vi "MGCC_StaEst_opal_RT_convertPnode.vi"(10 "cluster":T1) -> (2 "P_node":T1)   [LabVIEW 2016]
doc: "-----------------------------------------------------------------------------------------------------------------------\nCopyright <2019> <The University of Tennessee at Knoxville and the University of Tennessee Research Foundation>\nThis software is released under BSD-3 \nhttps://opensource.org/licenses/BSD-3-Clause \nAdditional license options available at https://utrf.tennessee.edu/industry/sample-agreements/\n-----------------------------------------------------------------------------------------------------------------------"
uses:
  Model Management/Global_MdlMgmt.vi
  <vilib>/imath/engines/lvmath2/RunTimeEngine/IndexRead/NIMS M($,S).vi
  <instcachedir>/0/NIMS M($,S)_3E5749BBB62E49528D4765A77F1F6D98.lvgen/NIMS M($,S)_3E5749BBB62E49528D4765A77F1F6D98_001.vi
  <vilib>/imath/engines/lvmath2/RunTimeEngine/BuiltInFunctions/length/NIMS_length(GV).vi
  <instcachedir>/0/NIMS_length(GV)_08A3D13377FD4E4B96F5795FBF3698FA.lvgen/NIMS_length(GV)_08A3D13377FD4E4B96F5795FBF3698FA_001.vi
  <vilib>/imathl/engines/lvmath/Functions/Error Handling/Create Error.vi
  <vilib>/imath/engines/lvmath2/RunTimeEngine/RangeToken/NIMS_Range_R3 - Integer.vi
  <instcachedir>/0/NIMS_Range_R3 - Integer_A435E2FF893B4C718FD5055FE39FE2F6.lvgen/NIMS_Range_R3 - Integer_A435E2FF893B4C718FD5055FE39FE2F6_000.vi
  <vilib>/imath/engines/lvmath2/RunTimeEngine/CommandStatement/MC_CommandStatement_break.vi
  <vilib>/imath/engines/lvmath2/RunTimeEngine/IndexRead/NIMS V(S).vi
  <instcachedir>/0/NIMS V(S)_0488751826AF41519A22953C041130DC.lvgen/NIMS V(S)_0488751826AF41519A22953C041130DC_000.vi
  <vilib>/imath/engines/lvmath2/RunTimeEngine/IndexReplace/NIMS M(S,$)=V.vi
  <instcachedir>/0/NIMS M(S,$)=V_BCCFA522A894489B8FA760383D74A164.lvgen/NIMS M(S,$)=V_BCCFA522A894489B8FA760383D74A164_001.vi
  <instcachedir>/0/NIMS M($,S)_3E5749BBB62E49528D4765A77F1F6D98.lvgen/NIMS M($,S)_3E5749BBB62E49528D4765A77F1F6D98_000.vi
  <instcachedir>/0/NIMS_length(GV)_08A3D13377FD4E4B96F5795FBF3698FA.lvgen/NIMS_length(GV)_08A3D13377FD4E4B96F5795FBF3698FA_000.vi
  <vilib>/imath/engines/lvmath2/RunTimeEngine/IndexRead/NIMS M(S,S).vi
  <instcachedir>/0/NIMS M(S,S)_AC51E74150A542F7991B9634C66F3096.lvgen/NIMS M(S,S)_AC51E74150A542F7991B9634C66F3096_000.vi
  <vilib>/imath/engines/lvmath2/RunTimeSupport/NIMS_Error if Not Equal.vi
  <instcachedir>/0/NIMS_Error if Not Equal_43252A79AD05436189442EC0C5E5AB8A.lvgen/NIMS_Error if Not Equal_43252A79AD05436189442EC0C5E5AB8A_000.vi
  <vilib>/imath/engines/lvmath2/RunTimeEngine/ErrorHandling/NIMS_Create Error From Enums.vi
  <vilib>/imath/engines/lvmath2/RunTimeEngine/IndexRead/NIMS M(S,$).vi
  <instcachedir>/0/NIMS M(S,$)_F24F360562DE41D8BE234322A2E15C65.lvgen/NIMS M(S,$)_F24F360562DE41D8BE234322A2E15C65_001.vi
  <vilib>/imath/engines/lvmath2/RunTimeEngine/NodeEndStatement/NIMS_NodeEndStatement_Output.vi
  <instcachedir>/0/NIMS_NodeEndStatement_Output_53EC0D466D134D7ABD903AC30B43404B.lvgen/NIMS_NodeEndStatement_Output_53EC0D466D134D7ABD903AC30B43404B_003.vi
  <vilib>/imath/engines/lvmath2/RunTimeEngine/ErrorHandling/NIMS_Finalize Error.vi
panel:
  out "Slack_bus":dbl[](array[numeric])
  out "element":dbl
  out "f_MGCC_OnliTopoIden_EnergizedMatrix":dbl[](array[numeric])
  out "error out":errorcluster
  out "p_node 2":cdb[][](array[numeric])
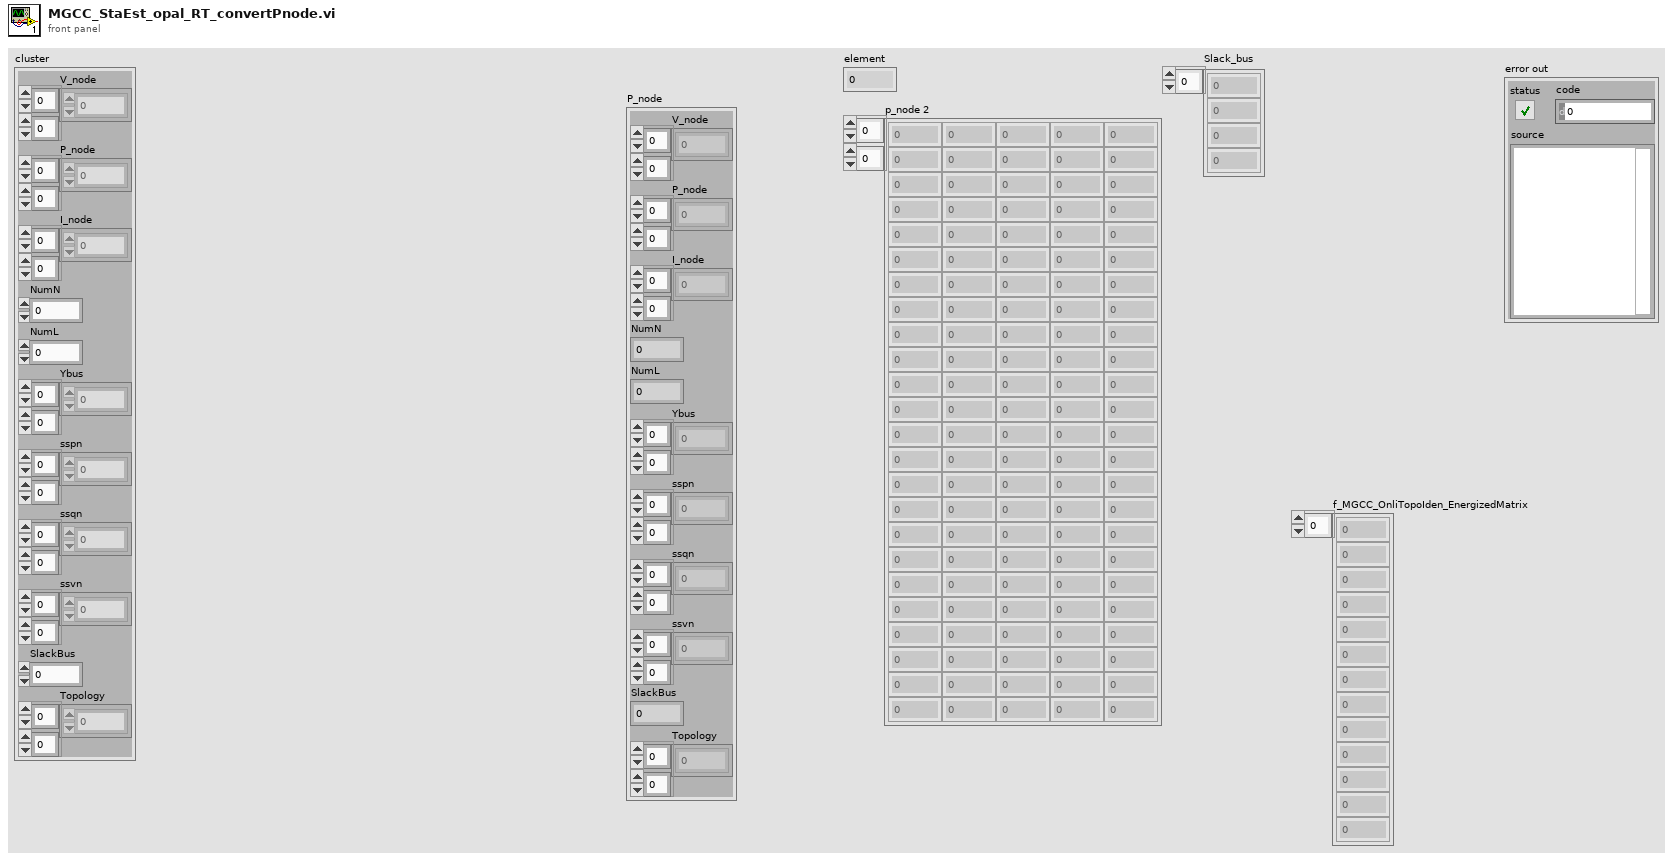
[diagram p1: front panel]
types:
  T1 = cluster{"V_node":cdb[][], "P_node":cdb[][], "I_node":cdb[][], "NumN":dbl, "NumL":dbl, "Ybus":cdb[][], "sspn":dbl[][], "ssqn":dbl[][], "ssvn":dbl[][], "SlackBus":dbl, "Topology":dbl[][]}
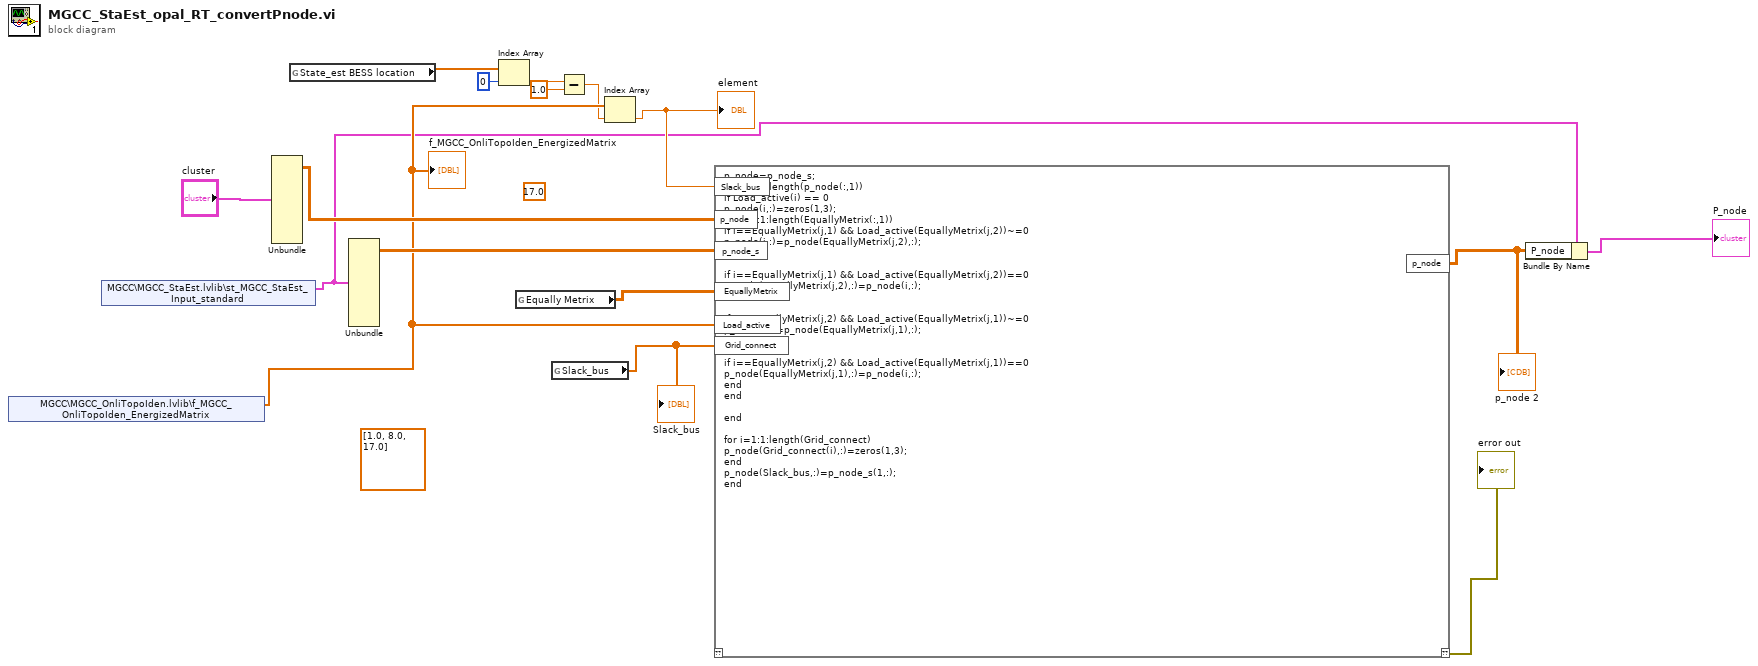
[diagram p0: block diagram]
diagram:
  (unwired) dbl[] [1.0, 8.0, 17.0] ("Grid_connect")
  (unwired) 17.0 ("Slack_bus")
  n1 = shared-variable "MGCC\\MGCC_OnliTopoIden.lvlib\\f_MGCC_OnliTopoIden_EnergizedMatrix"() -> (w13:dbl[])  [unwired: 1 in, 1 out]
  "f_MGCC_OnliTopoIden_EnergizedMatrix" <- w13
  n2 = shared-variable "MGCC\\MGCC_StaEst.lvlib\\st_MGCC_StaEst_Input_standard"() -> (w2:T1)  [unwired: 1 in, 1 out]
  n3 = Unbundle("cluster") -> ("P_node"=w16:cdb[][])  [unwired: 10 out]
  n4 = global read "Global_MdlMgmt.vi" "State_est BESS location"() -> (w11:dbl[])
  n5 = Unbundle(w2) -> ("P_node"=w15:cdb[][])  [unwired: 10 out]
  n6 = Index Array(array=w11, index=0) -> (element=w5:dbl)
  n7 = global read "Global_MdlMgmt.vi" "Equally Metrix"() -> (w9:dbl[][])
  n8 = global read "Global_MdlMgmt.vi" "Slack_bus"() -> (w8:dbl[])
  "Slack_bus" <- w8
  n9 = Subtract(x=w5, y=1.0) -> (x-y=w3:dbl)
  n10 = Index Array(array=w13, index=w3) -> (element=w7:dbl)
  "element" <- w7
  n11 = mathscript code="p_node=p_node_s;\nfor i=1:1:length(p_node(:,1))\nif Load_active(i) == 0\np_node(i,:)=zeros(1,3);\nfor j=1:1:length(EquallyMetrix(:,1))\nif i==EquallyMetrix(j,1) && Load_active(EquallyMetrix(j,2))~=0\np_node(i,:)=p_node(EquallyMetrix(j,2),:);\nend\n\nif i==EquallyMetrix(j,1) && Load_active(EquallyMetrix(j,2))==0\np_node(EquallyMetrix(j,2),:)=p_node(i,:);\nend\n\nif i==EquallyMetrix(j,2) && Load_active(EquallyMetrix(j,1))~=0\np_node(i,:)=p_node(EquallyMetrix(j,1),:);\nend\n\nif i==EquallyMetrix(j,2) && Load_active(EquallyMetrix(j,1))==0\np_node(EquallyMetrix(j,1),:)=p_node(i,:);\nend\nend\n\nend\n\nfor i=1:1:length(Grid_connect)\np_node(Grid_connect(i),:)=zeros(1,3);\nend\np_node(Slack_bus,:)=p_node_s(1,:);\nend"("p_node"=w16, "p_node_s"=w15, "EquallyMetrix"=w9, "Load_active"=w13, "Slack_bus"=w7, "Grid_connect"=w8) -> ("??"=→"error out":errorcluster, "p_node"=w12:cdb[][])  [unwired: 1 in]
  "p_node 2" <- w12
  n12 = Bundle By Name(cluster=w2, "P_node"=w12) -> (→"P_node":T1)
